vi "Read Calibration path.vi"(8 "error in (no error)":errorcluster caption="entrée d'erreur (pas d'erreur)", 11 "Detector en entrée":refnum<class "Detector.lvclass">) -> (0 "error out":errorcluster caption="sortie d'erreur", 2 "Calibration path":path, 3 "Detector en sortie":refnum<class "Detector.lvclass">)   [LabVIEW 2015, in "Detector.lvclass"]
uses:
  Detector.lvclass
  Detector.lvclass/Detector.ctl
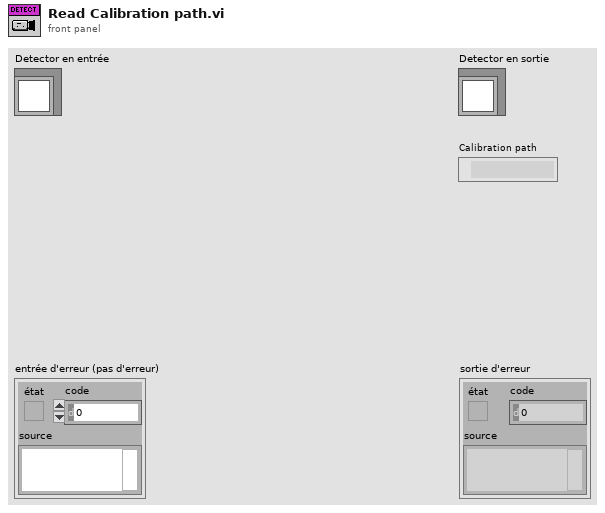
[diagram p1: front panel]
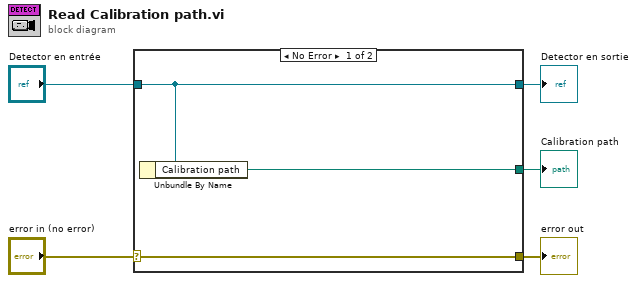
[diagram p0: block diagram]
diagram:
  n1 = case shown="No Error" "error in (no error)" {
    selector: "error in (no error)" -> [w8 w9]
    tunnel: [w8 w9] -> w4
    tunnel: [w7 w10] -> w2
    tunnel: "Detector en entrée" -> [w7 w10]
    tunnel: [w6 _] -> w1
    frame No Error {
      n2 = Unbundle By Name(w7) -> ("Calibration path"=w6:path)
    }
    frame Error {
    }
  }
  "error out" <- w4
  "Detector en sortie" <- w2
  "Calibration path" <- w1
